vi "PhaseSpace.vi"() -> ()   [LabVIEW 2011]
uses:
  ctrOWLMarker.ctl
  ctrCommonFlags.ctl
  ctrSetsFlags.ctl
  <vilib>/Platform/TimedLoop/XDataNode/timing_clust.ctl
  <vilib>/Platform/TimedLoop/XDataNode/nitl_modes.ctl
  <vilib>/Platform/TimedLoop/XDataNode/wakeup.ctl
  <vilib>/Platform/TimedLoop/XDataNode/XDataNode.xnode
  C:/Program Files/Phasespace/libowlsock.dll
  <vilib>/Platform/TimedLoop/XDataNode/XDNodeRunTimeDep.lvlib
panel:
  in  "stop":bool
  out "markers obtained (err: <0)":u16
  out "markers":T1[](array[typedef])
  out "connected to server?":bool
  in  "server address":string="192.168.0.101"
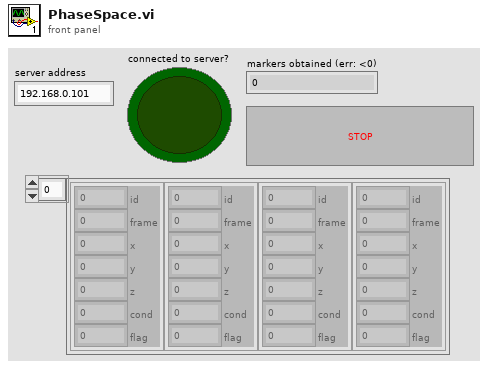
[diagram p1: front panel]
types:
  T1 = typedef "ctrOWLMarker.ctl" = cluster{"id":i32, "frame":i32, "x":sgl, "y":sgl, "z":sgl, "cond":sgl, "flag":u32}
  T2 = enum16{"open", "open or create", "create or replace", "create", "open (read-only)"}
  T3 = typedef "XDNodeRunTimeDep.lvlib/timing_clust.ctl" = cluster{"Expected End [f-1]":u64, "Actual End [f-1]":u64, "Finished Late? [f-1]":bool, "Expected End [i-1]":u64, "Actual End [i-1]":u64, "Finished Late? [i-1]":bool, "Expected Start [i]":u64, "Actual Start [i]":u64, "Expected Start [f]":u64, "Actual Start [f]":u64, "Source Name":string, "Structure Name":string, "Period":i64, "Deadline":i64, "Offset":i64, "Start":i64, "Priority":i32, "Timeout":i32, "Mode":T4, "Wakeup Reason":T5, "Error":errorcluster, "Source Type":string, "Secondary Source Type":string, "Global End Time":u64, "Global Start Time":u64, "Frame Duration":u64, "Iteration Duration":u64, "Assigned CPU":i32, "I/O Scan Engine Mode":u32}
  T4 = typedef "XDNodeRunTimeDep.lvlib/nitl_modes.ctl" = enum32{"No Change", "Process missed periods, maintain original phase", "Discard missed periods, maintain original phase", "Process missed periods, ignore original phase", "Discard missed periods, ignore original phase"}
  T5 = typedef "XDNodeRunTimeDep.lvlib/wakeup.ctl" = enum32{"Normal", "Aborted", "Asynchronous wakeup", "Timing source error", "Timed loop error", "Timeout"}
  T6 = typedef "ctrCommonFlags.ctl" = u16
  T7 = typedef "ctrSetsFlags.ctl" = u16
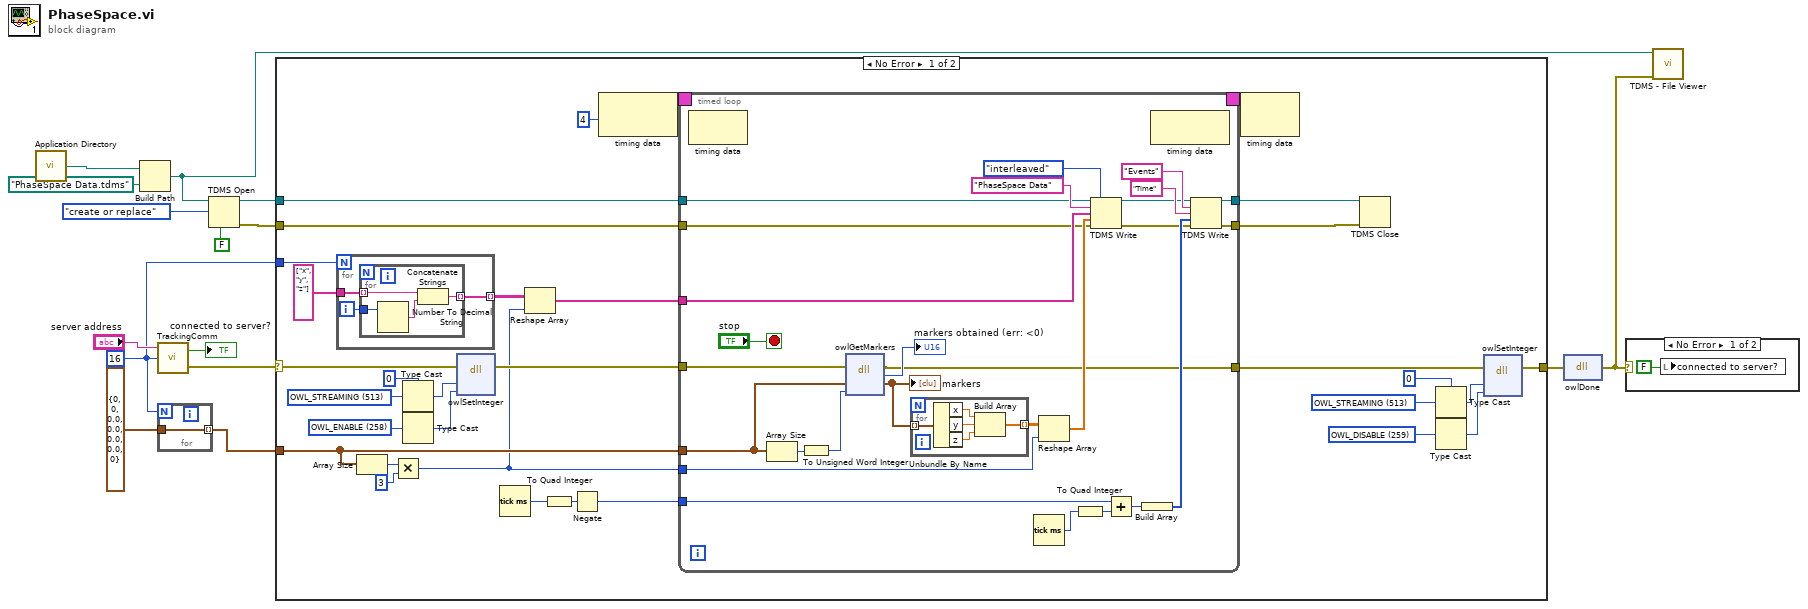
[diagram p0: block diagram]
diagram:
  w7 = 16 ("marker tally (default: 32)")
  n1 = call <vilib>:"Application Directory.vi"() -> ("Application Directory"=w9:path)
  n2 = Build Path(base path=w9, name or relative path=path "PhaseSpace Data.tdms" ("file path")) -> (appended path=w1:path)
  n3 = call "TrackingComm.vi"("marker tally (default: 32)"=w7, "server address"="server address") -> ("error out"=w6:errorcluster, "connected to server?"=→"connected to server?":bool)  [unwired: 1 in]
  n4 = for {
    N: w7 -> [_]
    tunnel: T1 {"id"=0, "frame"=0, "x"=0.0, "y"=0.0, "z"=0.0, "cond"=0.0, "flag"=0} -> [w16]
    tunnel: [w16] -> w5 mode=indexing
  }
  n5 = TDMS Open(6:FALSE ("disable buffering? (T)"), 10:T2."create or replace" ("operation"), 11:w1) -> (0:w4:errorcluster, 3:w8:refnum<k34>)  [unwired: 3 in]
  n6 = case shown="No Error" w6 {
    selector: w6 -> [w35 w94]
    tunnel: w8 -> [w37 _]
    tunnel: w7 -> [w36 _]
    tunnel: w5 -> [w34 _]
    tunnel: w4 -> [w31 _]
    tunnel: [w21 w94] -> w2
    frame No Error {
      w25 = u16 0
      w24 = T6 259 items=["OWL_CREATE"=256, "OWL_DESTROY"=257, "OWL_ENABLE"=258, "OWL_DISABLE"=259] ("Common flages")
      w23 = T7 513 items=["OWL_FREQUENCY"=512, "OWL_STREAMING"=513, "OWL_INTERPOLATION"=514, "OWL_BUTTONS"=528, "OWL_MARKERS"=529, "OWL_RIGIDS"=530, "OWL_COMMDATA"=544, "OWL_TIMESTAMP"=545, "OWL_PLANES"=672, "OWL_DETECTORS"=673, "OWL_IMAGES"=674, "OWL_TRANSFORM"=49664] ("Sets flags")
      w48 = u16 0
      w45 = T6 258 items=["OWL_CREATE"=256, "OWL_DESTROY"=257, "OWL_ENABLE"=258, "OWL_DISABLE"=259] ("Common flages")
      w44 = T7 513 items=["OWL_FREQUENCY"=512, "OWL_STREAMING"=513, "OWL_INTERPOLATION"=514, "OWL_BUTTONS"=528, "OWL_MARKERS"=529, "OWL_RIGIDS"=530, "OWL_COMMDATA"=544, "OWL_TIMESTAMP"=545, "OWL_PLANES"=672, "OWL_DETECTORS"=673, "OWL_IMAGES"=674, "OWL_TRANSFORM"=49664] ("Sets flags")
      n7 = for {
        N: w36 -> [_]
        tunnel: string[] ["x", "y", "z"] -> [w89]
        tunnel: [w87] -> w40 mode=indexing
        i -> [w88]
        n8 = for {
          tunnel: w89 -> [w93] mode=indexing
          tunnel: w88 -> [w92]
          tunnel: [w90] -> w87 mode=indexing
          n9 = Number To Decimal String(number=w92) -> (decimal integer string=w91:string)  [unwired: 1 in]
          n10 = Concatenate Strings(w93, w91) -> (w90:string)
        }
      }
      n11 = Array Size(array=w34) -> (size(s)=w43:i32)
      n12 = Multiply(x=w43, y=3) -> (x*y=w18:i32)
      n13 = Type Cast(type=w48, x=w44) -> (*(type *) &x=w47:u16)
      n14 = Type Cast(type=w48, x=w45) -> (*(type *) &x=w46:u16)
      n15 = dll-call lib="C:/Program Files/Phasespace/libowlsock.dll" fn="owlSetInteger"(error in=w35, "pname"=w47, "param"=w46) -> (error out=w33:errorcluster)  [unwired: 4 in, 2 out]
      n16 = Tick Count (ms)() -> (millisecond timer value=w39:u32)
      n17 = Reshape Array(w40, w18) -> (w32:string[])
      n18 = To Quad Integer(1:w39) -> (0:w38:i64)
      n19 = Negate(x=w38) -> (-x=w30:i64)
      n20 = node-c288(i64 4 ("Period")) -> (w20:T3)
      n21 = timed-loop {
        tunnel: w37 -> [w67]
        tunnel: w34 -> [w66]
        tunnel: w33 -> [w65]
        tunnel: w32 -> [w64]
        tunnel: w31 -> [w63]
        tunnel: w30 -> [w56]
        tunnel: [w53] -> w29
        tunnel: [w52] -> w28
        tunnel: [w51] -> w22
        timing: w20 -> [_]
        timing-out: [_] -> w19
        tunnel: w18 -> [w49]
        stop <- "stop" stop-if-true
        n22 = node-c288() -> ()  [unwired: 1 in, 1 out]
        n23 = Array Size(array=w66) -> (size(s)=w74:i32)
        n24 = To Unsigned Word Integer(number=w74) -> (unsigned 16bit integer=w75:u16)
        n25 = dll-call lib="C:/Program Files/Phasespace/libowlsock.dll" fn="owlGetMarkers"(error in=w65, "markers"=w66, "count"=w75) -> (error out=w51:errorcluster, "return type"=→"markers obtained (err: <0)":u16, "markers"=w71:T1[])  [unwired: 3 in, 1 out]
        "markers" <- w71
        n26 = for {
          tunnel: w71 -> [w82] mode=indexing
          tunnel: [w78] -> w72 mode=indexing
          n27 = Unbundle By Name(w82) -> ("x"=w81:sgl, "y"=w80:sgl, "z"=w79:sgl)
          n28 = Build Array(w81, w80, w79) -> (w78:sgl[])
        }
        n29 = Tick Count (ms)() -> (millisecond timer value=w61:u32)
        n30 = Reshape Array(w72, w49) -> (w69:sgl[])
        n31 = To Quad Integer(1:w61) -> (0:w62:i64)
        n32 = TDMS Write(0:w67, 1:enum16{"decimated", "interleaved"}."interleaved" ("data layout (0:decimated)"), 5:"PhaseSpace Data" ("group name"), 7:w64, 9:w69, 11:w63) -> (4:w54:refnum<k34>, 15:w55:errorcluster)  [unwired: 2 out]
        n33 = Add(x=w56, y=w62) -> (x+y=w60:i64)
        n34 = Build Array(w60) -> (w57:i64[])
        n35 = node-c288() -> ()  [unwired: 1 in, 1 out]
        n36 = TDMS Write(0:w54, 5:"Events" ("group name"), 7:"Time" ("channel name"), 9:w57, 11:w55) -> (4:w53:refnum<k34>, 15:w52:errorcluster)  [unwired: 1 in, 2 out]
      }
      n37 = node-c288(w19) -> ()  [unwired: 1 out]
      n38 = TDMS Close(8:w28, 11:w29) -> ()  [unwired: 2 out]
      n39 = Type Cast(type=w25, x=w23) -> (*(type *) &x=w26:u16)
      n40 = Type Cast(type=w25, x=w24) -> (*(type *) &x=w27:u16)
      n41 = dll-call lib="C:/Program Files/Phasespace/libowlsock.dll" fn="owlSetInteger"(error in=w22, "pname"=w26, "param"=w27) -> (error out=w21:errorcluster)  [unwired: 4 in, 2 out]
    }
    frame Error {
    }
  }
  n42 = dll-call lib="C:/Program Files/Phasespace/libowlsock.dll" fn="owlDone"(error in=w2) -> (error out=w3:errorcluster)  [unwired: 2 in, 2 out]
  n43 = case shown="No Error" w3 {
    frame No Error {
      n44 = local write "connected to server?"(FALSE) -> ()
    }
    frame Error {
    }
  }
  n45 = call <vilib>:"TDMS - File Viewer.vi"("error in (no error)"=w3, "file path"=w1) -> ()  [unwired: 6 out]
